vi "Config Motors.vi"(11 "Primay Current Limit (80A)":dbl=80.0) -> ()   [LabVIEW 2018]
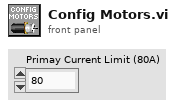
[diagram p1: front panel]
types:
  T1 = typedef "WPI_MotorControlDeviceRef.ctl" = cluster{"DeviceStatus":errorcluster, "Type":T2, "PWM":cluster{"PWM Channel":T3, "DeadBand":T4}, "CAN":cluster{"Device Number":u8, "SetOutput VI Ref":variant, "GetOutput VI Ref":variant, "Enable VI Ref":variant, "Disable VI Ref":variant, "Data":variant}, "Invert":bool, "DIO PWM":cluster{"PWM \"Enable\" Channel":T3, "DIOChannel":T5, "PWM Rate":dbl}}
  T2 = typedef "WPI_MotorControlType.ctl" = enum16{"PWM", "CAN", "DIO PWM"}
  T3 = typedef "FPGA_DIOPWMChannel.ctl" = enum8{"PWM 0", "PWM 1", "PWM 2", "PWM 3", "PWM 4", "PWM 5", "PWM 6", "PWM 7", "PWM 8", "PWM 9", "PWM MXP 0", "PWM MXP 1", "PWM MXP 2", "PWM MXP 3", "PWM MXP 4", "PWM MXP 5", "PWM MXP 6", "PWM MXP 7", "PWM MXP 8", "PWM MXP 9", "Invalid"}
  T4 = typedef "WPI_PWMDeadband.ctl" = cluster{"Name":string, "maxPositivePwm":i32, "minPositivePwm":i32, "centerPwm":i32, "maxNegativePwm":i32, "minNegativePwm":i32, "angularRange":u16}
  T5 = typedef "FPGA_DIOChannel.ctl" = enum8{"DIO 0", "DIO 1", "DIO 2", "DIO 3", "DIO 4", "DIO 5", "DIO 6", "DIO 7", "DIO 8", "DIO 9", "DIO MXP 0", "DIO MXP 1", "DIO MXP 2", "DIO MXP 3", "DIO MXP 4", "DIO MXP 5", "DIO MXP 6", "DIO MXP 7", "DIO MXP 8", "DIO MXP 9", "DIO MXP 10", "DIO MXP 11", "DIO MXP 12", "DIO MXP 13", "DIO MXP 14", "DIO MXP 15", "SPI Port CS1", "SPI Port CS2", "SPI Port CS3", "SPI Port MISO", "SPI Port MOSI", "Invalid"}
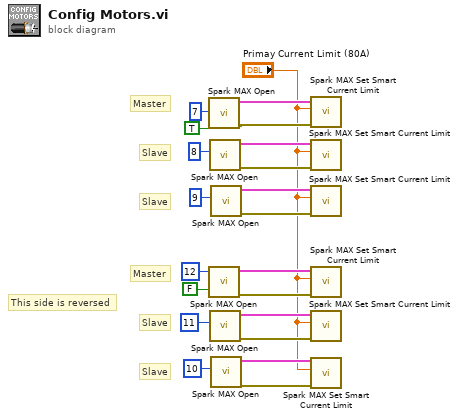
[diagram p0: block diagram]
diagram:
  # "This side is reversed"
  # "Slave"
  # "Slave"
  # "Master"
  # "Slave"
  # "Slave"
  # "Master"
  n1 = call <vilib>:"Spark MAX Open.vi"("Invert"=TRUE, "Device Number"=u8 7) -> ("error out"=w12:errorcluster, "MotorControlDeviceRef"=w13:T1)  [unwired: 8 in]
  n2 = call <vilib>:"Spark MAX Open.vi"("Invert"=FALSE, "Device Number"=u8 12) -> ("error out"=w6:errorcluster, "MotorControlDeviceRef"=w7:T1)  [unwired: 8 in]
  n3 = call <vilib>:"Spark MAX Open.vi"("Device Number"=u8 8) -> ("error out"=w10:errorcluster, "MotorControlDeviceRef"=w11:T1)  [unwired: 9 in]
  n4 = call <vilib>:"Spark MAX Open.vi"("Device Number"=u8 11) -> ("error out"=w4:errorcluster, "MotorControlDeviceRef"=w5:T1)  [unwired: 9 in]
  n5 = call <vilib>:"Spark MAX Open.vi"("Device Number"=u8 9) -> ("error out"=w8:errorcluster, "MotorControlDeviceRef"=w9:T1)  [unwired: 9 in]
  n6 = call <vilib>:"Spark MAX Open.vi"("Device Number"=u8 10) -> ("error out"=w2:errorcluster, "MotorControlDeviceRef"=w3:T1)  [unwired: 9 in]
  n7 = call <vilib>:"Spark MAX Set Smart Current Limit.vi"("error in (no error)"=w12, "Primay Current Limit (80A)"="Primay Current Limit (80A)", "MotorControlDeviceRef in"=w13) -> ()  [unwired: 7 in, 2 out]
  n8 = call <vilib>:"Spark MAX Set Smart Current Limit.vi"("error in (no error)"=w10, "Primay Current Limit (80A)"="Primay Current Limit (80A)", "MotorControlDeviceRef in"=w11) -> ()  [unwired: 7 in, 2 out]
  n9 = call <vilib>:"Spark MAX Set Smart Current Limit.vi"("error in (no error)"=w8, "Primay Current Limit (80A)"="Primay Current Limit (80A)", "MotorControlDeviceRef in"=w9) -> ()  [unwired: 7 in, 2 out]
  n10 = call <vilib>:"Spark MAX Set Smart Current Limit.vi"("error in (no error)"=w6, "Primay Current Limit (80A)"="Primay Current Limit (80A)", "MotorControlDeviceRef in"=w7) -> ()  [unwired: 7 in, 2 out]
  n11 = call <vilib>:"Spark MAX Set Smart Current Limit.vi"("error in (no error)"=w4, "Primay Current Limit (80A)"="Primay Current Limit (80A)", "MotorControlDeviceRef in"=w5) -> ()  [unwired: 7 in, 2 out]
  n12 = call <vilib>:"Spark MAX Set Smart Current Limit.vi"("error in (no error)"=w2, "Primay Current Limit (80A)"="Primay Current Limit (80A)", "MotorControlDeviceRef in"=w3) -> ()  [unwired: 7 in, 2 out]
